vi "_FPGA_Timebase.vi"(1 "HalfPeriod":u16=1) -> (0 "Clk_out":bool)   [LabVIEW 2018]
uses:
  <instrlib>/_niInstr/Basic Elements/v1/FPGA/niInstr Basic Elements v1 FPGA.lvlib
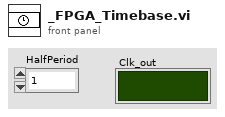
[diagram p1: front panel]
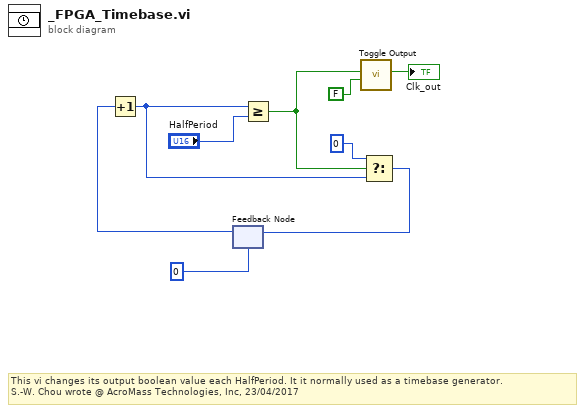
[diagram p0: block diagram]
diagram:
  # "This vi changes its output boolean value each HalfPeriod. It it normally used as a timebase generator.\nS.-W. Chou wrote @ AcroMass Technologies, Inc, 23/04/2017"
  n1 = feedback #1(u16 0) -> (w7:u16)
  n2 = Increment(x=w7) -> (x+1=w6:u16)
  n3 = Greater Or Equal?(x=w6, y="HalfPeriod") -> (x >= y?=w3:bool)
  n4 = call <instrlib>:"Toggle Output.vi"("clear"=FALSE, "toggle"=w3) -> ("output"=→"Clk_out":bool)  [unwired: 9 in]
  n5 = Select(t=u16 0, s=w3, f=w6) -> (s? t:f=w4:u16)
  n6 = feedback-in #1(w4) -> ()
